vi "QueueManager__slk_QSM-PC (String).vi"(6 "action (back)":enum16{"Back", "Front", "Replace"}(ring), 7 "queue in":refnum<queue>, 8 "error in (no error)":errorcluster, 10 "elements":cluster{"State":string, "Data":variant}[](array[cluster])) -> (0 "error out":errorcluster)   [LabVIEW 2016, in "QSM-PC (String).lvlib"]
doc: "Manages the methods of equeuing and error handling.\n\n<b>Equeue Method:</b>\nEnqueue to the back of queue\nEnqueue to the front of queue\nReplace the elements of queue\n<b>Error Handling State:</b>\nError Handling"
uses:
  Library/QSM-PC (String).lvlib
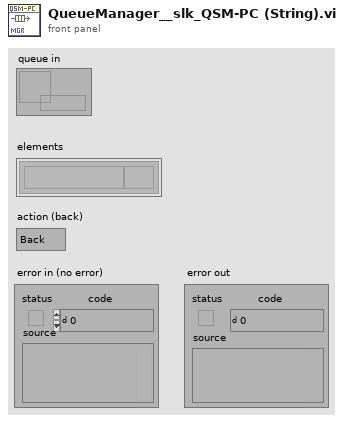
[diagram p1: front panel]
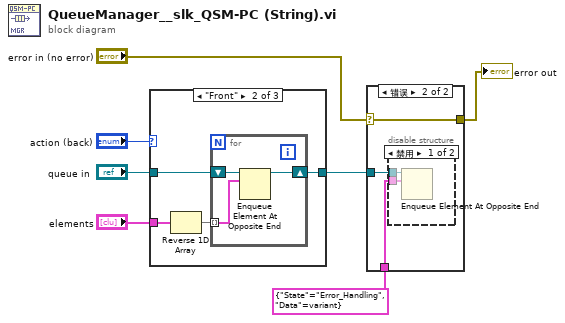
[diagram p0: block diagram]
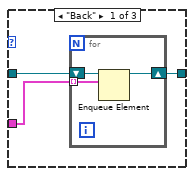
[diagram p4: hidden frame]
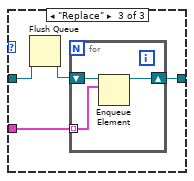
[diagram p5: hidden frame]
diagram:
  n1 = case shown="\"Front\"" "action (back)" {
    tunnel: "queue in" -> [w10 w17 w22]
    tunnel: "elements" -> [w9 w16 w23]
    tunnel: [w8 w15 w24] -> w5
    frame "Back" {
      n2 = for {
        tunnel: w9 -> [w12] mode=indexing
        shift-right: [w11] -> w8
        shift-left: w10 -> [w13]
        n3 = Enqueue Element(queue=w13, element=w12) -> (queue out=w11:refnum<queue>)  [unwired: 1 in, 3 out]
      }
    }
    frame "Front" {
      n4 = Reverse 1D Array(array=w16) -> (reversed array=w14:cluster{"State":string, "Data":variant}[])
      n5 = for {
        tunnel: w14 -> [w19] mode=indexing
        shift-right: [w18] -> w15
        shift-left: w17 -> [w20]
        n6 = Enqueue Element At Opposite End(queue=w20, element=w19) -> (queue out=w18:refnum<queue>)  [unwired: 1 in, 3 out]
      }
    }
    frame "Replace" {
      n7 = Flush Queue(queue=w22) -> (queue out=w21:refnum<queue>)  [unwired: 1 in, 2 out]
      n8 = for {
        tunnel: w23 -> [w26] mode=indexing
        shift-right: [w25] -> w24
        shift-left: w21 -> [w27]
        n9 = Enqueue Element(queue=w27, element=w26) -> (queue out=w25:refnum<queue>)  [unwired: 1 in, 3 out]
      }
    }
  }
  n10 = case shown="错误" "error in (no error)" {
    selector: "error in (no error)" -> [w28 w29]
    tunnel: w5 -> [_ w31]
    tunnel: cluster{"State":string, "Data":variant} {"State"="Error_Handling", "Data"=variant} ("Element") -> [_ w30]
    tunnel: [w28 w29] -> w1
    frame No Error {
    }
    frame Error {
      n11 = disable-structure shown="禁用" {
        disable-tunnel: w31 -> [w33 _]
        disable-tunnel: w30 -> [w32 _]
        frame Disabled {
          n12 = Enqueue Element At Opposite End(queue=w33, element=w32) -> ()  [unwired: 1 in, 4 out]
        }
        frame Enabled {
        }
      }
    }
  }
  "error out" <- w1
